vi "detSetpointFromProfile.vi"(8 "error in (no error)":errorcluster, 11 "Model in":refnum<class "Model.lvclass">) -> (0 "error out":errorcluster, 3 "Model out":refnum<class "Model.lvclass">)   [LabVIEW 2015]
uses:
  ApplicationElements/TestMonitor/TestMonitor.lvclass
  Model.lvclass
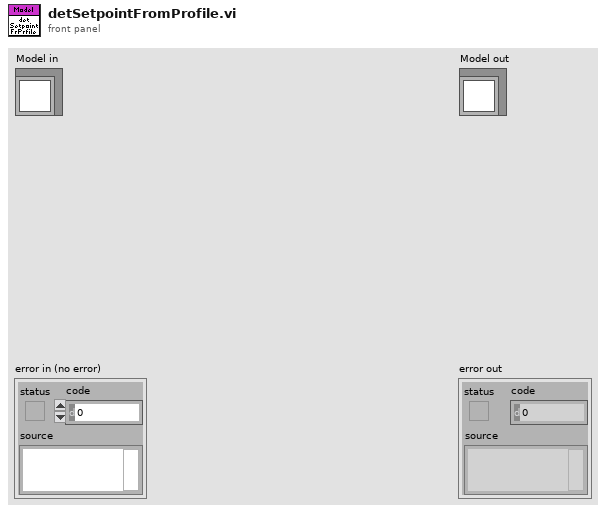
[diagram p1: front panel]
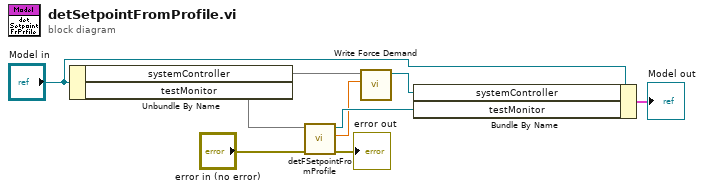
[diagram p0: block diagram]
diagram:
  n1 = Unbundle By Name("Model in") -> ("systemController"=w3, "testMonitor"=w9)
  n2 = call "detFSetpointFromProfile.vi"("error in (no error)"="error in (no error)", "TestMonitor in"=w9) -> ("error out"=→"error out":errorcluster, "forceSetpoint"=w1:dbl[unit], "TestMonitor out"=w8:refnum<class "TestMonitor.lvclass">)  [unwired: 7 in]
  n3 = call "Write Force Demand.vi"("Force Demand"=w1, "SystemController in"=w3) -> ("SystemController out"=w2:refnum<class "SystemController.lvclass">)  [unwired: 9 in]
  n4 = Bundle By Name(cluster="Model in", "systemController"=w2, "testMonitor"=w8) -> (→"Model out":cluster{})
